vi "一体站单参数流程质控自动启动.vi"(6 "CODMn量程切换":enum32{"H", "L", "AUTO"}(ring)=enum."AUTO", 8 "总磷量程切换":enum32{"H", "L", "AUTO"}(ring)=enum."AUTO", 9 "总氮量程切换":enum32{"H", "L", "AUTO"}(ring)=enum."AUTO", 10 "氨氮量程切换":enum32{"H", "L", "AUTO"}(ring)=enum."AUTO", 11 "参数":T1={"是否启用仪器"=FALSE, "CODMn"={"启动测量模式"={"测量模式"=enum."水样测量"}, "确定按钮"=TRUE}, "启动模块"={"氨氮"=FALSE, "总磷"=FALSE, "总氮"=FALSE, "CODMn"=FALSE, "CODCr"=FALSE}, "常规启动"=FALSE, "直接启动"=FALSE}) -> ()   [LabVIEW 2016]
panel:
  out "枚举":enum16{"初始化", "采配水启动", "等待", "配水", "排水", "结束"}(ring)
  out "枚举 2":enum16{"初始化", "采配水启动", "等待", "配水", "排水", "结束"}(ring)
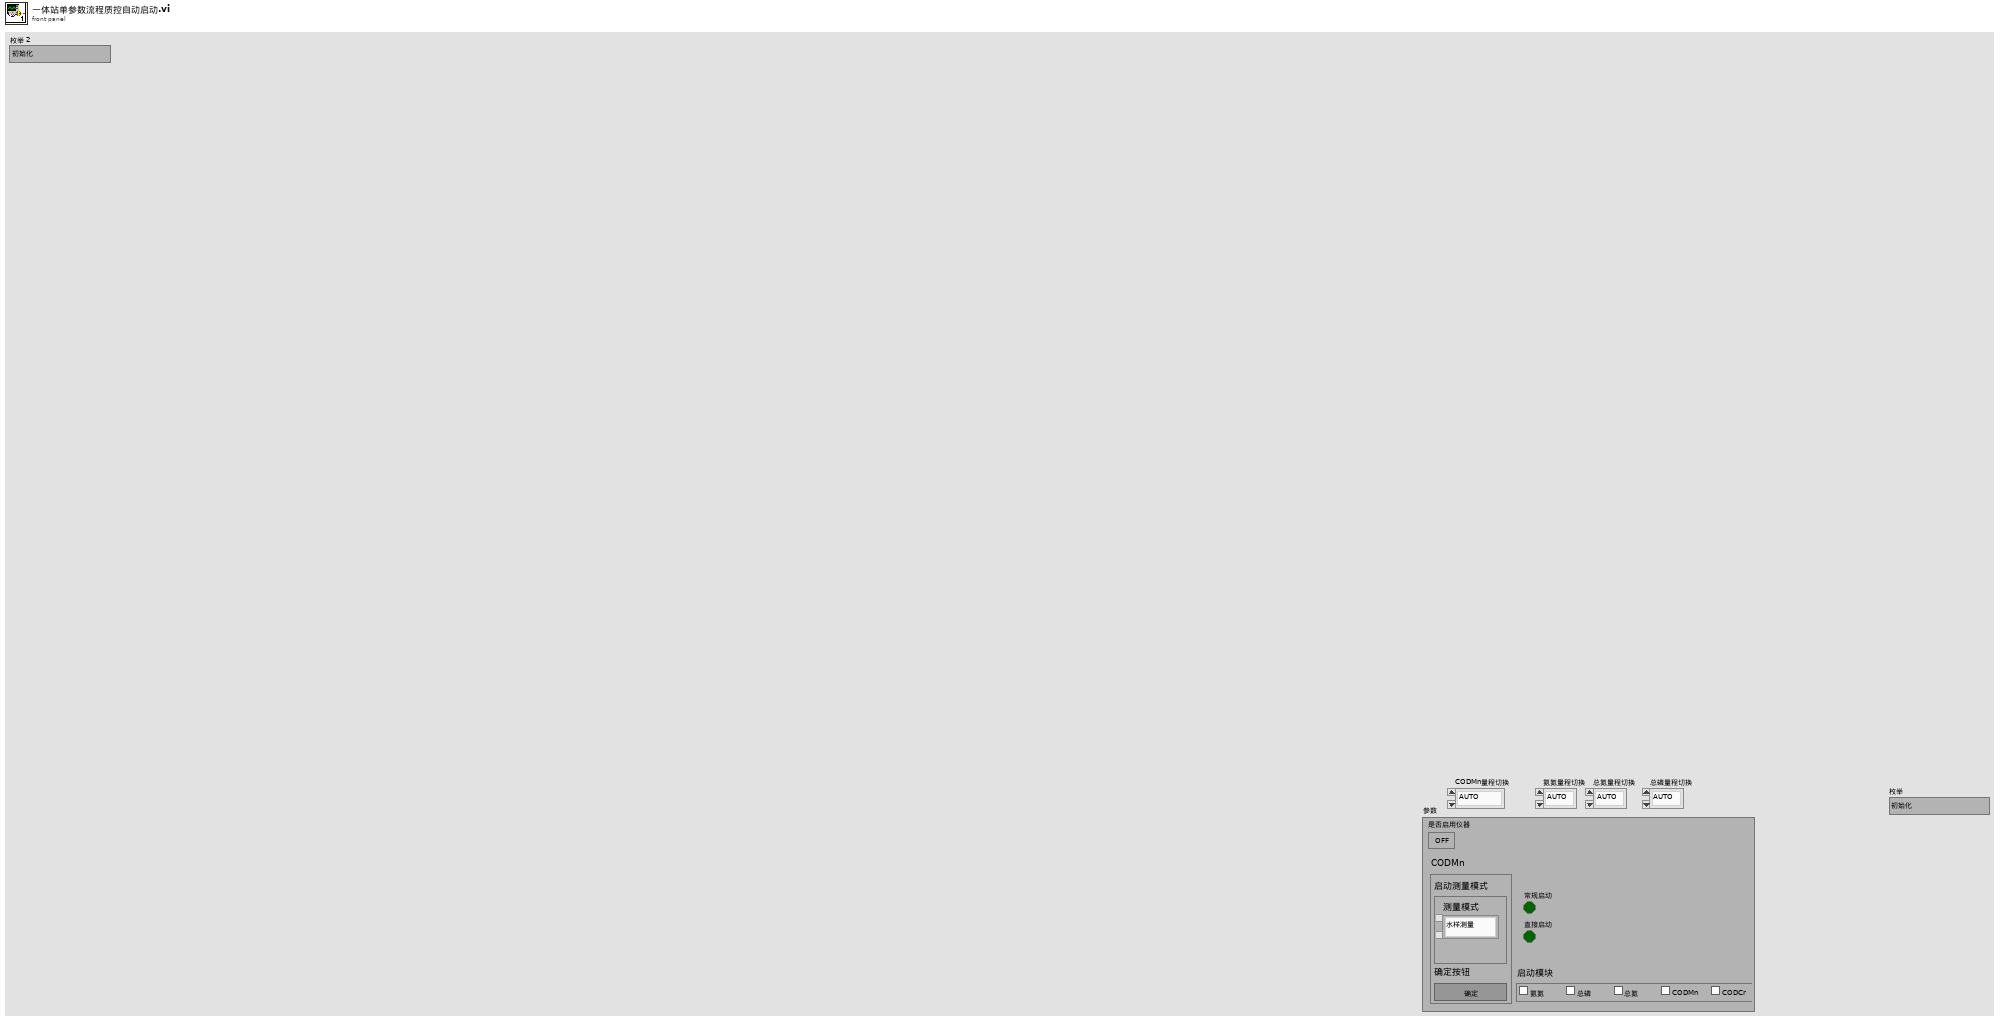
[diagram p1: front panel]
types:
  T1 = cluster{"是否启用仪器":bool, "CODMn":cluster{"启动测量模式":cluster{"测量模式":enum16{"水样测量", "标样核查", "加标回收", "平行样", "校零", "校标"}}, "确定按钮":bool}, "启动模块":cluster{"氨氮":bool, "总磷":bool, "总氮":bool, "CODMn":bool, "CODCr":bool}, "常规启动":bool, "直接启动":bool}
  T2 = cluster{"命令":string, cluster{"starting address":u16, "holding register value":u16}}
  T3 = cluster{"R0":i16, "R1":i16, "R2":i16, "R3":i16, "R4":i16, "R5":i16, "R6":i16, "R7":i16, "R8":i16, "R9":i16, "R10":i16, "R11":i16, "R12":i16, "R13":i16, "R14":i16, "R15":i16, "R16":i16, "R17":i16, "R18":i16, "R19":i16, "R20":i16, "R21":i16, "R22":i16, "R23":i16, "R24":i16, "R25":i16, "R26":i16, "R27":i16, "R28":i16, "R29":i16, "R30":i16, "R31":i16, "R32":i16, "R33":i16, "R34":i16, "R35":i16, "R36":i16, "R37":i16, "R38":i16, "R39":i16, "R40":i16, "R41":i16, "R42":i16, "R43":i16, "R44":i16, "R45":i16, "R46":i16, "R47":i16, "R48":i16, "R49":i16, "R50":i16, "R51":i16, "R52":i16, "R53":i16, "R54":i16, "R55":i16, "R56":i16}
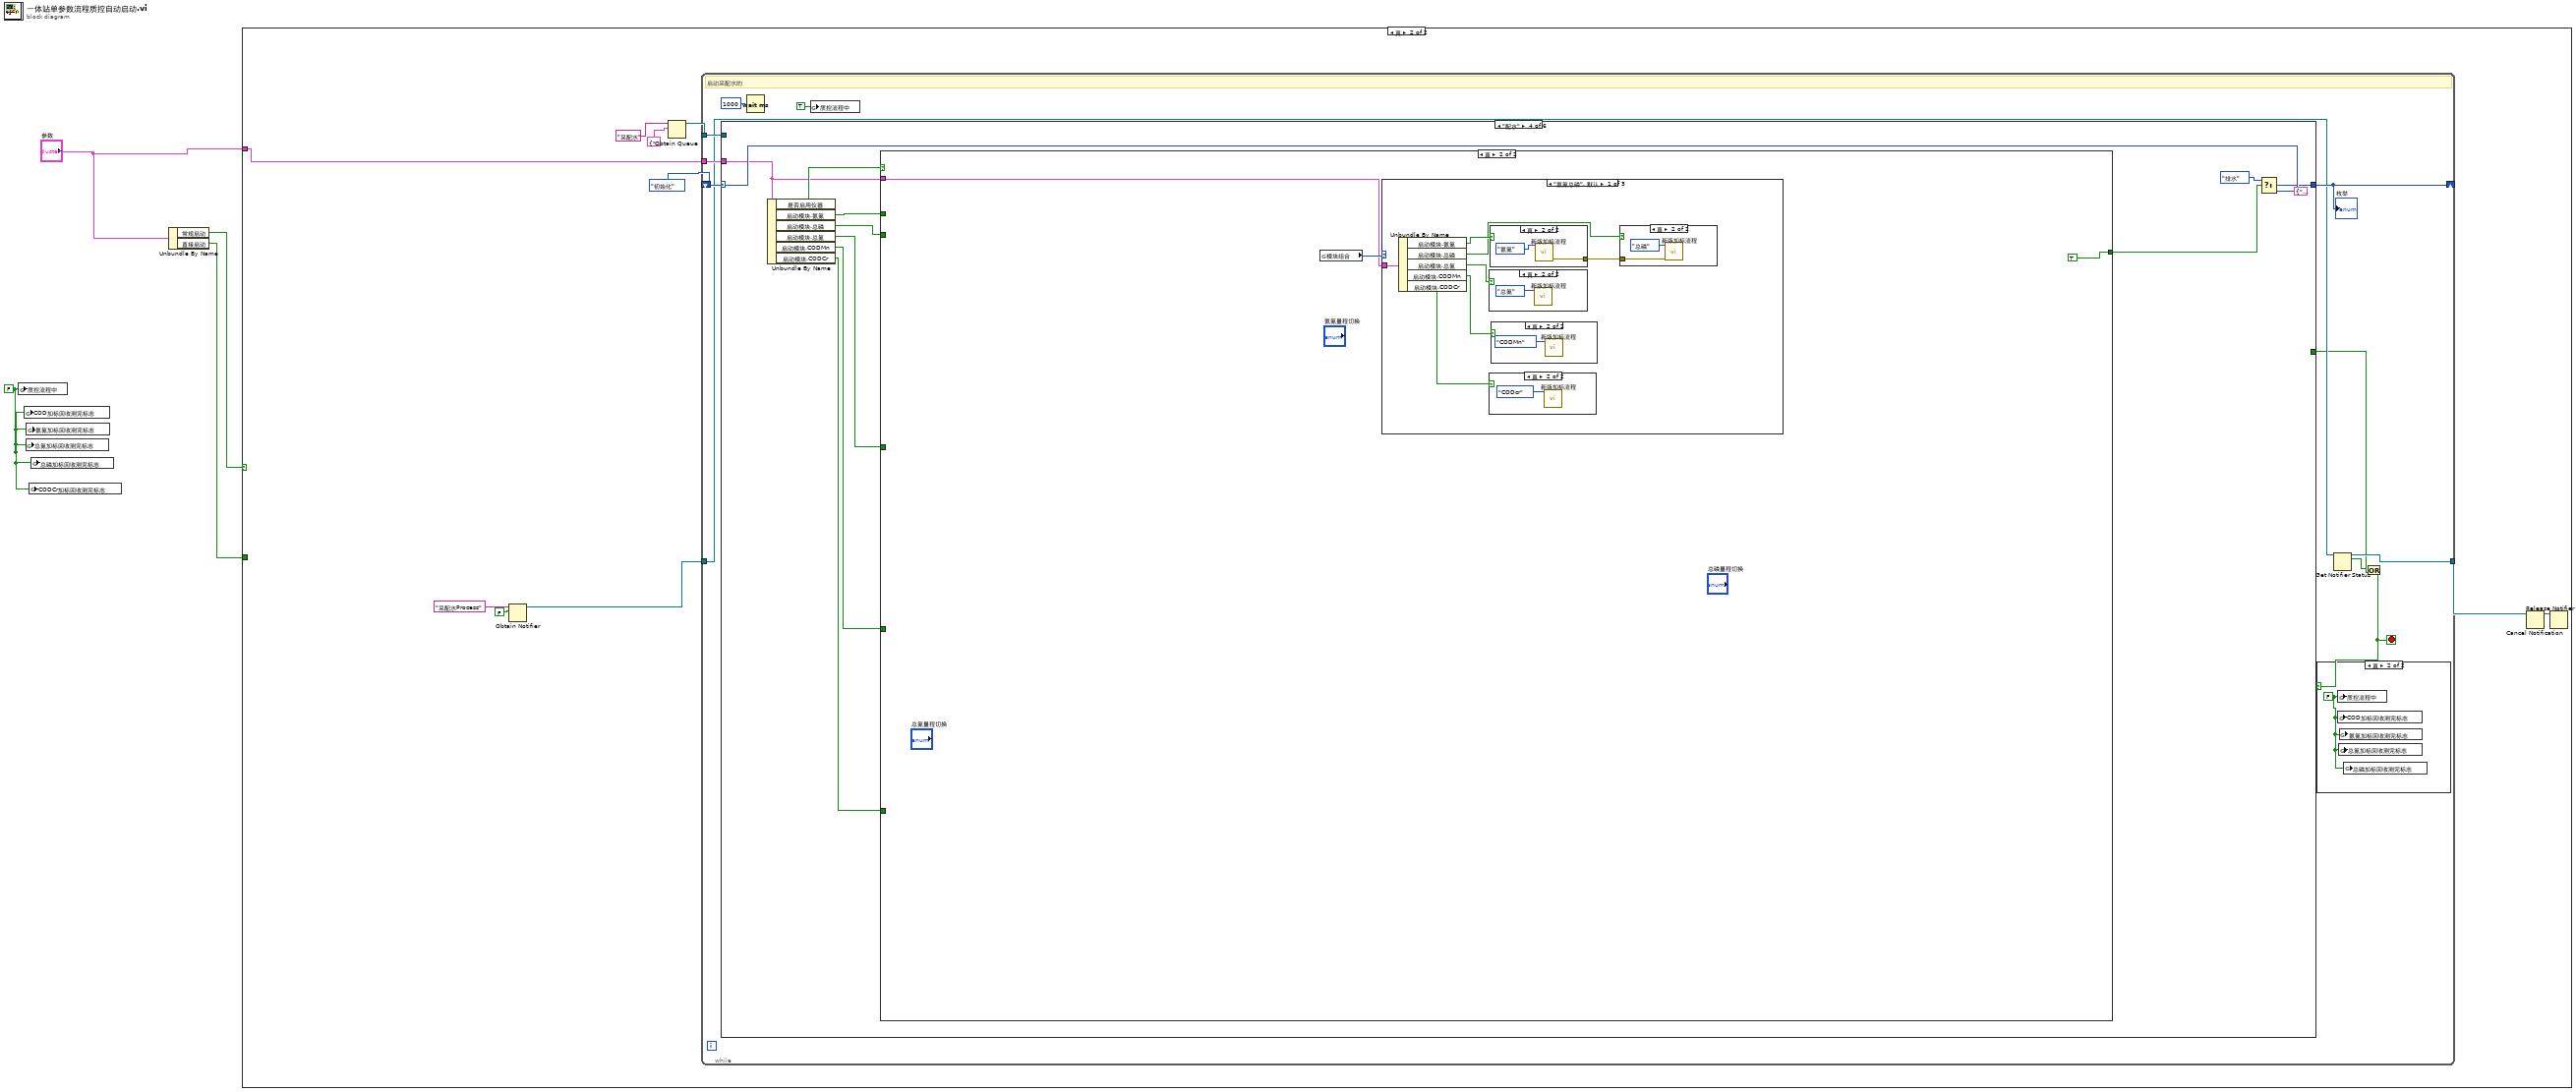
[diagram p0: block diagram]
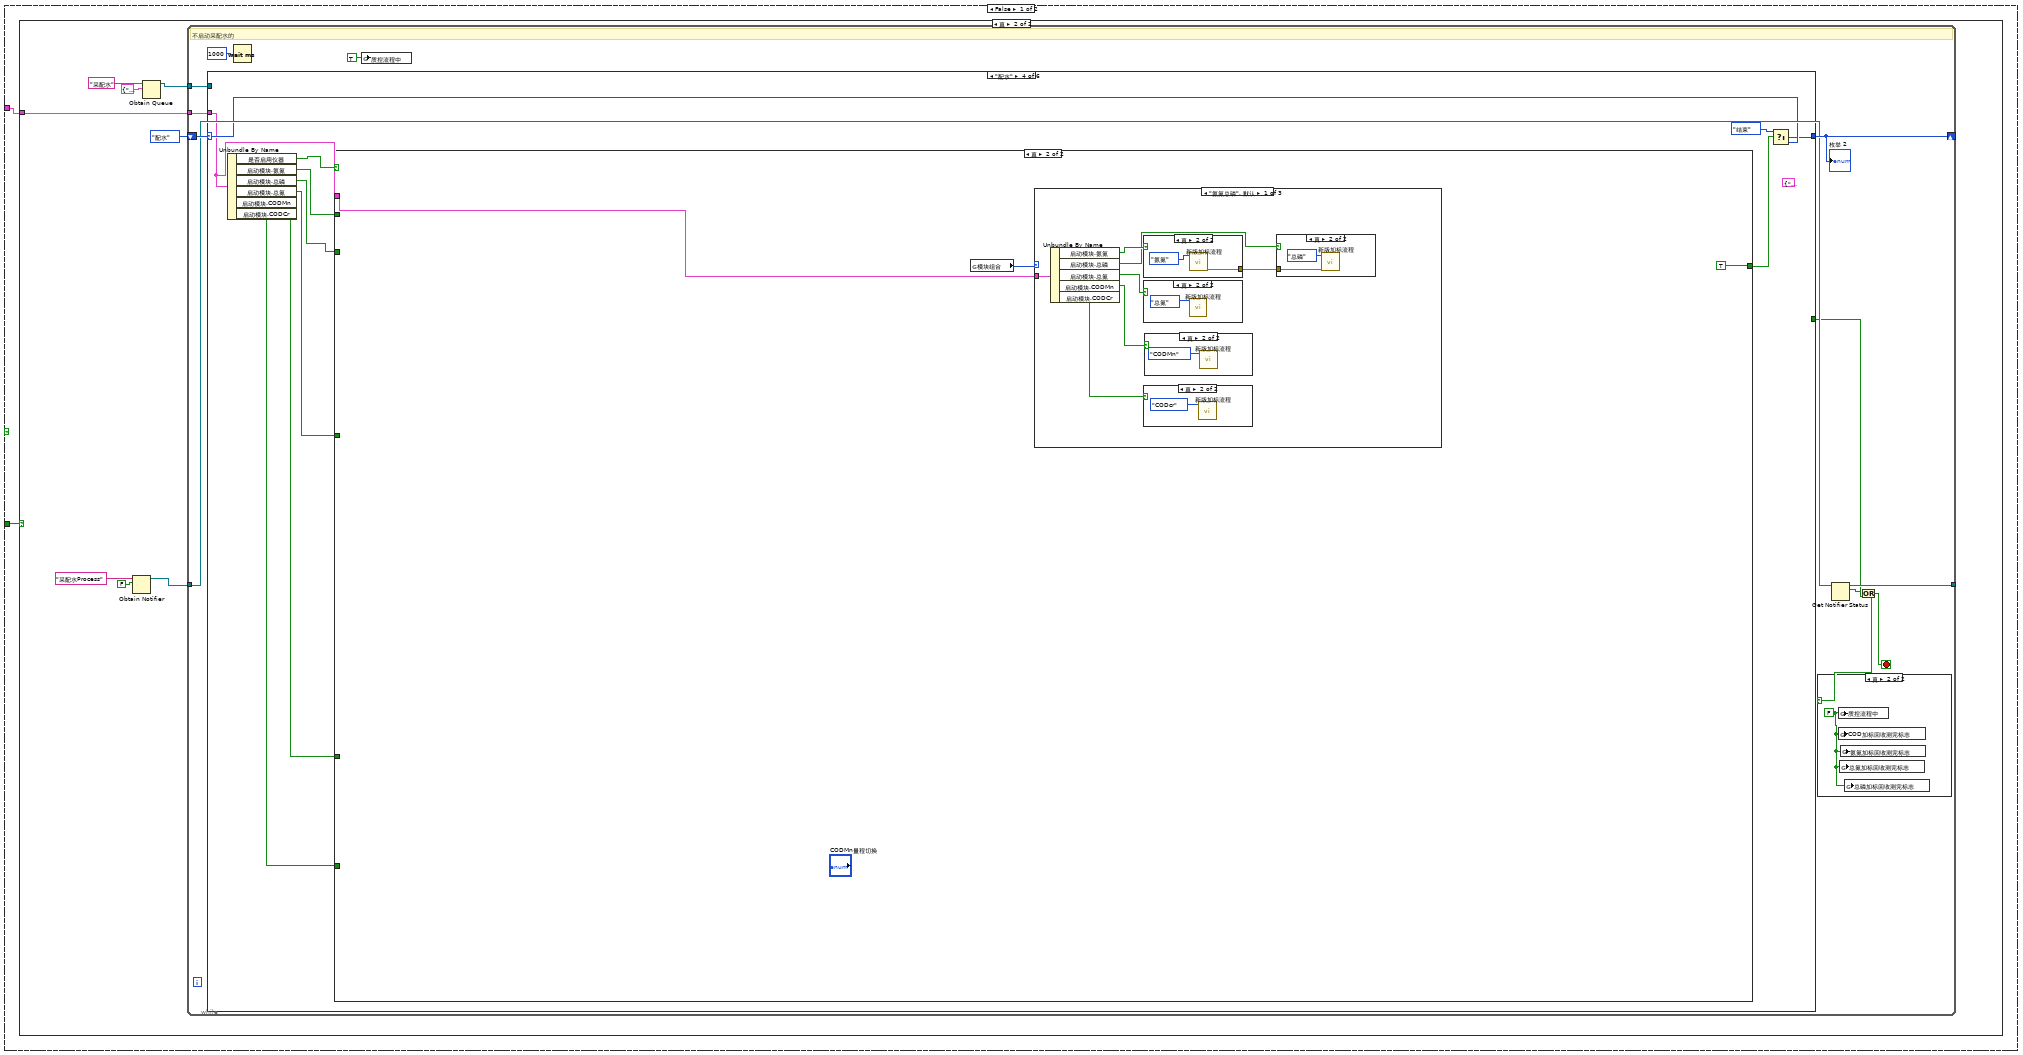
[diagram p2: hidden frame]
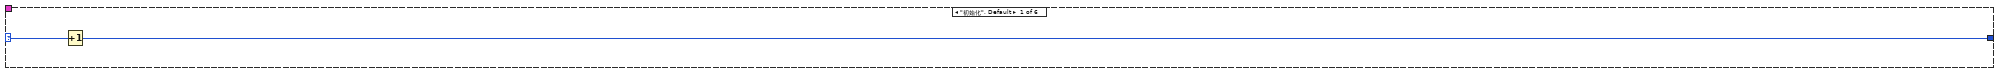
[diagram p5: hidden frame]
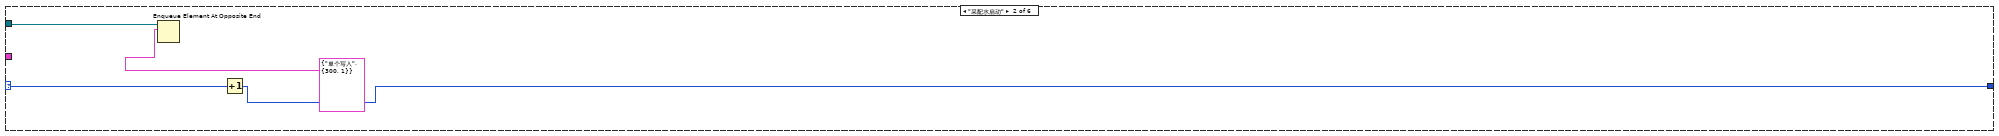
[diagram p6: hidden frame]
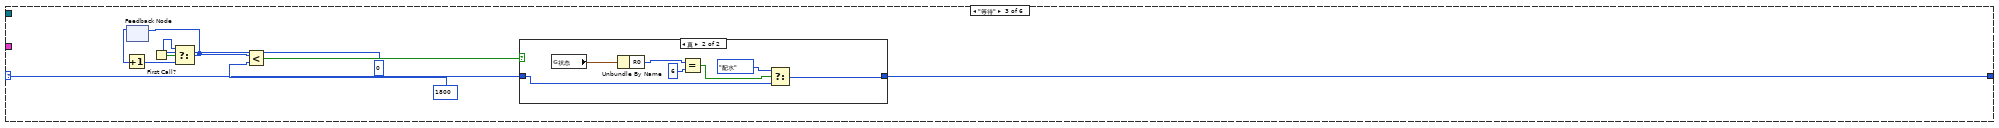
[diagram p7: hidden frame]
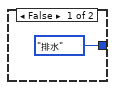
[diagram p8: hidden frame]
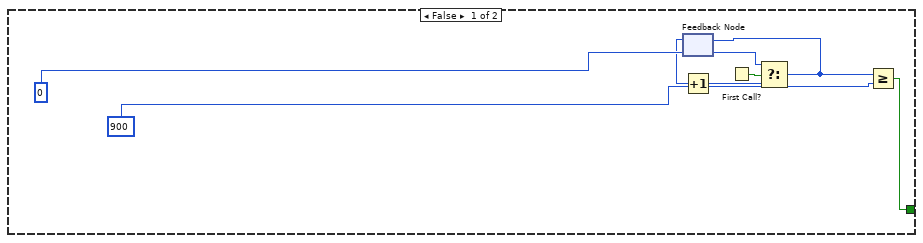
[diagram p9: hidden frame]
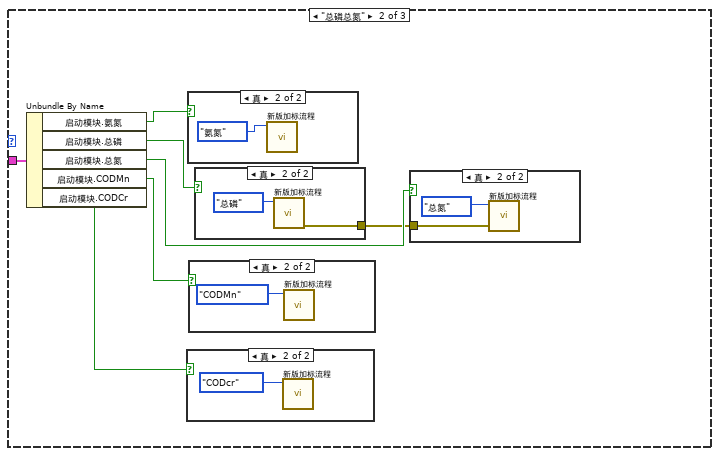
[diagram p15: hidden frame]
diagram:
  w1 = FALSE ("质控流程中")
  n1 = global write "质控测完标志全局 1.vi" "质控流程中"(w1) -> ()
  n2 = global write "质控测完标志全局 1.vi" "COD加标回收测完标志"(w1) -> ()
  n3 = global write "质控测完标志全局 1.vi" "总氮加标回收测完标志"(w1) -> ()
  n4 = global write "质控测完标志全局 1.vi" "氨氮加标回收测完标志"(w1) -> ()
  n5 = global write "质控测完标志全局 1.vi" "CODCr加标回收测完标志"(w1) -> ()
  n6 = global write "质控测完标志全局 1.vi" "总磷加标回收测完标志"(w1) -> ()
  n7 = Unbundle By Name("参数") -> ("常规启动"=w3:bool, "直接启动"=w2:bool)
  n8 = case shown="真" w3 {
    tunnel: "参数" -> [w5 w117]
    tunnel: w2 -> [w6 _]
    frame False {
      n9 = case shown="真" w6 {
        tunnel: w5 -> [_ w13]
        frame False {
        }
        frame True {
          n10 = Obtain Notifier(name (unnamed)="采配水Process" ("名称（未命名）"), notification data type=FALSE) -> (notifier out=w7:refnum<notifier>)  [unwired: 2 in, 2 out]
          n11 = Obtain Queue(name (unnamed)="采配水" ("名称（未命名）"), element data type=cluster{"命令":string, "数据":variant} {"命令"="", "数据"=variant}) -> (queue out=w10:refnum<queue>)  [unwired: 3 in, 2 out]
          n12 = while {
            tunnel: w10 -> [w25]
            shift-right: [w23] -> _
            shift-left: enum16{"初始化", "采配水启动", "等待", "配水", "排水", "结束"}."配水" ("枚举") -> [w24]
            tunnel: w13 -> [w21]
            tunnel: w7 -> [w20]
            tunnel: [w19] -> _
            stop <- w16 stop-if-true
            # "不启动采配水的"
            n13 = case shown="\"配水\"" w24 {
              selector: w24 -> [w28 w30 w39 w59 w111 w116]
              tunnel: w25 -> [_ w31 _ _ w112 _]
              tunnel: [w27 w29 w38 w58 w110 w115] -> w23
              tunnel: [_ _ _ _ _ TRUE] -> w18
              tunnel: w21 -> [_ _ _ w50 _ _]
              frame "初始化", Default {
                n14 = Increment(x=w28) -> (x+1=w27:enum16{"初始化", "采配水启动", "等待", "配水", "排水", "结束"})
              }
              frame "采配水启动" {
                n15 = Enqueue Element At Opposite End(queue=w31, element=T2 {"命令"="单个写入", {"starting address"=300, "holding register value"=1}} ("元素")) -> ()  [unwired: 2 in, 3 out]
                n16 = Increment(x=w30) -> (x+1=w29:enum16{"初始化", "采配水启动", "等待", "配水", "排水", "结束"})
              }
              frame "等待" {
                n17 = feedback #1() -> (w35:i32)  [unwired: 1 in]
                n18 = Increment(x=w35) -> (x+1=w34:i32)
                n19 = First Call?() -> (First Call?: T/F=w36:bool)
                n20 = Select(t=0, s=w36, f=w34) -> (s? t:f=w33:i32)
                n21 = feedback-in #1(w33) -> ()
                n22 = Less?(x=w33, y=1800) -> (x < y?=w40:bool)
                n23 = case shown="真" w40 {
                  tunnel: w39 -> [_ w45]
                  tunnel: [enum16{"初始化", "采配水启动", "等待", "配水", "排水", "结束"}."排水" ("枚举") w44] -> w38
                  frame False {
                  }
                  frame True {
                    n24 = global read "与采配水交互全局.vi" "状态"() -> (w43:T3)
                    n25 = Unbundle By Name(w43) -> ("R0"=w49:i16)
                    n26 = Equal?(x=w49, y=i16 6) -> (x = y?=w47:bool)
                    n27 = Select(t=enum16{"初始化", "采配水启动", "等待", "配水", "排水", "结束"}."配水" ("枚举"), s=w47, f=w45) -> (s? t:f=w44:enum16{"初始化", "采配水启动", "等待", "配水", "排水", "结束"})
                  }
                }
              }
              frame "配水" {
                (unwired) cluster{"命令":string, "data":variant} {"命令"="启动", "data"=variant(cluster{"站号":u16, "控制命令输出":u16[]} {"站号"=1, "控制命令输出"=[256, 0]})} ("元素")
                n28 = Unbundle By Name(w50) -> ("是否启用仪器"=w57:bool, "启动模块.氨氮"=w54:bool, "启动模块.总磷"=w55:bool, "启动模块.总氮"=w52:bool, "启动模块.CODMn"=w53:bool, "启动模块.CODCr"=w51:bool)
                n29 = case shown="真" w57 {
                  tunnel: [w61 TRUE] -> w56
                  tunnel: w55 -> [_ _]
                  tunnel: w54 -> [_ _]
                  tunnel: w53 -> [_ _]
                  tunnel: w52 -> [_ _]
                  tunnel: w51 -> [_ _]
                  tunnel: w50 -> [_ w69]
                  frame False {
                    n30 = feedback #2() -> (w65:i32)  [unwired: 1 in]
                    n31 = Increment(x=w65) -> (x+1=w64:i32)
                    n32 = First Call?() -> (First Call?: T/F=w66:bool)
                    n33 = Select(t=0, s=w66, f=w64) -> (s? t:f=w62:i32)
                    n34 = feedback-in #2(w62) -> ()
                    n35 = Greater Or Equal?(x=w62, y=900) -> (x >= y?=w61:bool)
                  }
                  frame True {
                    n36 = global read "断电保存全局.vi" "模块组合"() -> (w70:enum16{"氨氮总磷", "总磷总氮", "氨氮、总磷、总氮"})
                    n37 = case shown="\"氨氮总磷\", 默认" w70 {
                      tunnel: w69 -> [w77 w88 w104]
                      frame "氨氮总磷", Default {
                        n38 = Unbundle By Name(w77) -> ("启动模块.氨氮"=w76:bool, "启动模块.总磷"=w74:bool, "启动模块.总氮"=w73:bool, "启动模块.CODMn"=w72:bool, "启动模块.CODCr"=w71:bool)
                        n39 = case shown="真" w73 {
                          frame False {
                          }
                          frame True {
                            n40 = call "新版加标流程.vi"("参数"=enum16{"氨氮", "总磷", "总氮", "CODMn", "CODcr"}."总氮") -> ()  [unwired: 10 in, 1 out]
                          }
                        }
                        n41 = case shown="真" w71 {
                          frame False {
                          }
                          frame True {
                            n42 = call "新版加标流程.vi"("参数"=enum16{"氨氮", "总磷", "总氮", "CODMn", "CODcr"}."CODcr") -> ()  [unwired: 10 in, 1 out]
                          }
                        }
                        n43 = case shown="真" w76 {
                          tunnel: [_ w83] -> w75
                          frame False {
                          }
                          frame True {
                            n44 = call "新版加标流程.vi"("参数"=enum16{"氨氮", "总磷", "总氮", "CODMn", "CODcr"}."氨氮") -> ("error out"=w83:errorcluster)  [unwired: 10 in]
                          }
                        }
                        n45 = case shown="真" w72 {
                          frame False {
                          }
                          frame True {
                            n46 = call "新版加标流程.vi"("参数"=enum16{"氨氮", "总磷", "总氮", "CODMn", "CODcr"}."CODMn") -> ()  [unwired: 10 in, 1 out]
                          }
                        }
                        n47 = case shown="真" w74 {
                          tunnel: w75 -> [_ w81]
                          frame False {
                          }
                          frame True {
                            n48 = call "新版加标流程.vi"("error in (no error)"=w81, "参数"=enum16{"氨氮", "总磷", "总氮", "CODMn", "CODcr"}."总磷") -> ()  [unwired: 9 in, 1 out]
                          }
                        }
                      }
                      frame "总磷总氮" {
                        n49 = Unbundle By Name(w88) -> ("启动模块.氨氮"=w91:bool, "启动模块.总磷"=w87:bool, "启动模块.总氮"=w86:bool, "启动模块.CODMn"=w90:bool, "启动模块.CODCr"=w89:bool)
                        n50 = case shown="真" w89 {
                          frame False {
                          }
                          frame True {
                            n51 = call "新版加标流程.vi"("参数"=enum16{"氨氮", "总磷", "总氮", "CODMn", "CODcr"}."CODcr") -> ()  [unwired: 10 in, 1 out]
                          }
                        }
                        n52 = case shown="真" w91 {
                          frame False {
                          }
                          frame True {
                            n53 = call "新版加标流程.vi"("参数"=enum16{"氨氮", "总磷", "总氮", "CODMn", "CODcr"}."氨氮") -> ()  [unwired: 10 in, 1 out]
                          }
                        }
                        n54 = case shown="真" w90 {
                          frame False {
                          }
                          frame True {
                            n55 = call "新版加标流程.vi"("参数"=enum16{"氨氮", "总磷", "总氮", "CODMn", "CODcr"}."CODMn") -> ()  [unwired: 10 in, 1 out]
                          }
                        }
                        n56 = case shown="真" w87 {
                          tunnel: [_ w96] -> w85
                          frame False {
                          }
                          frame True {
                            n57 = call "新版加标流程.vi"("参数"=enum16{"氨氮", "总磷", "总氮", "CODMn", "CODcr"}."总磷") -> ("error out"=w96:errorcluster)  [unwired: 10 in]
                          }
                        }
                        n58 = case shown="真" w86 {
                          tunnel: w85 -> [_ w94]
                          frame False {
                          }
                          frame True {
                            n59 = call "新版加标流程.vi"("error in (no error)"=w94, "参数"=enum16{"氨氮", "总磷", "总氮", "CODMn", "CODcr"}."总氮") -> ()  [unwired: 9 in, 1 out]
                          }
                        }
                      }
                      frame "氨氮、总磷、总氮" {
                        n60 = Unbundle By Name(w104) -> ("启动模块.氨氮"=w103:bool, "启动模块.总磷"=w102:bool, "启动模块.总氮"=w101:bool, "启动模块.CODMn"=w99:bool, "启动模块.CODCr"=w100:bool)
                        n61 = case shown="真" w102 {
                          frame False {
                          }
                          frame True {
                            n62 = call "新版加标流程.vi"("参数"=enum16{"氨氮", "总磷", "总氮", "CODMn", "CODcr"}."总磷") -> ()  [unwired: 10 in, 1 out]
                          }
                        }
                        n63 = case shown="真" w101 {
                          frame False {
                          }
                          frame True {
                            n64 = call "新版加标流程.vi"("参数"=enum16{"氨氮", "总磷", "总氮", "CODMn", "CODcr"}."总氮") -> ()  [unwired: 10 in, 1 out]
                          }
                        }
                        n65 = case shown="真" w103 {
                          frame False {
                          }
                          frame True {
                            n66 = call "新版加标流程.vi"("参数"=enum16{"氨氮", "总磷", "总氮", "CODMn", "CODcr"}."氨氮") -> ()  [unwired: 10 in, 1 out]
                          }
                        }
                        n67 = case shown="真" w99 {
                          frame False {
                          }
                          frame True {
                            n68 = call "新版加标流程.vi"("参数"=enum16{"氨氮", "总磷", "总氮", "CODMn", "CODcr"}."CODMn") -> ()  [unwired: 10 in, 1 out]
                          }
                        }
                        n69 = case shown="真" w100 {
                          frame False {
                          }
                          frame True {
                            n70 = call "新版加标流程.vi"("参数"=enum16{"氨氮", "总磷", "总氮", "CODMn", "CODcr"}."CODcr") -> ()  [unwired: 10 in, 1 out]
                          }
                        }
                      }
                    }
                  }
                }
                n71 = Select(t=enum16{"初始化", "采配水启动", "等待", "配水", "排水", "结束"}."结束" ("枚举"), s=w56, f=w59) -> (s? t:f=w58:enum16{"初始化", "采配水启动", "等待", "配水", "排水", "结束"})
              }
              frame "排水" {
                n72 = Enqueue Element At Opposite End(queue=w112, element=T2 {"命令"="单个写入", {"starting address"=303, "holding register value"=1}} ("元素")) -> ()  [unwired: 2 in, 3 out]
                n73 = Increment(x=w111) -> (x+1=w110:enum16{"初始化", "采配水启动", "等待", "配水", "排水", "结束"})
              }
              frame "结束" {
                n74 = Increment(x=w116) -> (x+1=w115:enum16{"初始化", "采配水启动", "等待", "配水", "排水", "结束"})
              }
            }
            "枚举 2" <- w23
            n75 = Wait (ms)(milliseconds to wait=u32 1000 ("等待时间（毫秒）")) -> ()  [unwired: 1 out]
            n76 = global write "质控测完标志全局 1.vi" "质控流程中"(TRUE ("质控流程中")) -> ()
            n77 = Get Notifier Status(notifier=w20) -> (notifier out=w19:refnum<notifier>, current notification=w17:bool)  [unwired: 1 in, 3 out]
            n78 = Or(x=w17, y=w18) -> (x .or. y?=w16:bool)
            n79 = case shown="真" w16 {
              frame False {
              }
              frame True {
                w26 = FALSE ("质控流程中")
                n80 = global write "质控测完标志全局 1.vi" "质控流程中"(w26) -> ()
                n81 = global write "质控测完标志全局 1.vi" "COD加标回收测完标志"(w26) -> ()
                n82 = global write "质控测完标志全局 1.vi" "总氮加标回收测完标志"(w26) -> ()
                n83 = global write "质控测完标志全局 1.vi" "氨氮加标回收测完标志"(w26) -> ()
                n84 = global write "质控测完标志全局 1.vi" "总磷加标回收测完标志"(w26) -> ()
              }
            }
          }
        }
      }
    }
    frame True {
      n85 = Obtain Notifier(name (unnamed)="采配水Process" ("名称（未命名）"), notification data type=FALSE) -> (notifier out=w120:refnum<notifier>)  [unwired: 2 in, 2 out]
      n86 = Obtain Queue(name (unnamed)="采配水" ("名称（未命名）"), element data type=cluster{"命令":string, "数据":variant} {"命令"="", "数据"=variant}) -> (queue out=w124:refnum<queue>)  [unwired: 3 in, 2 out]
      n87 = while {
        tunnel: w124 -> [w137]
        shift-right: [w135] -> _
        shift-left: enum16{"初始化", "采配水启动", "等待", "配水", "排水", "结束"}."初始化" ("枚举") -> [w136]
        tunnel: w117 -> [w133]
        tunnel: w120 -> [w132]
        tunnel: [w131] -> w119
        stop <- w128 stop-if-true
        # "启动采配水的"
        n88 = case shown="\"配水\"" w136 {
          selector: w136 -> [w140 w144 w153 w173 w225 w230]
          tunnel: w137 -> [_ w145 _ _ w226 _]
          tunnel: [w139 w143 w152 w172 w224 w229] -> w135
          tunnel: [_ _ _ _ _ TRUE] -> w130
          tunnel: w133 -> [_ _ _ w164 _ _]
          frame "初始化", Default {
            n89 = Increment(x=w140) -> (x+1=w139:enum16{"初始化", "采配水启动", "等待", "配水", "排水", "结束"})
          }
          frame "采配水启动" {
            n90 = Enqueue Element At Opposite End(queue=w145, element=T2 {"命令"="单个写入", {"starting address"=300, "holding register value"=1}} ("元素")) -> (queue out=w141:refnum<queue>)  [unwired: 2 in, 2 out]
            n91 = Increment(x=w144) -> (x+1=w143:enum16{"初始化", "采配水启动", "等待", "配水", "排水", "结束"})
            n92 = Enqueue Element At Opposite End(queue=w141, element=T2 {"命令"="单个写入", {"starting address"=303, "holding register value"=1}} ("元素")) -> ()  [unwired: 2 in, 3 out]
          }
          frame "等待" {
            n93 = feedback #3() -> (w149:i32)  [unwired: 1 in]
            n94 = Increment(x=w149) -> (x+1=w148:i32)
            n95 = First Call?() -> (First Call?: T/F=w150:bool)
            n96 = Select(t=0, s=w150, f=w148) -> (s? t:f=w147:i32)
            n97 = feedback-in #3(w147) -> ()
            n98 = Less?(x=w147, y=1800) -> (x < y?=w154:bool)
            n99 = case shown="真" w154 {
              tunnel: w153 -> [_ w159]
              tunnel: [enum16{"初始化", "采配水启动", "等待", "配水", "排水", "结束"}."排水" ("枚举") w158] -> w152
              frame False {
              }
              frame True {
                n100 = global read "与采配水交互全局.vi" "状态"() -> (w157:T3)
                n101 = Unbundle By Name(w157) -> ("R0"=w163:i16)
                n102 = Equal?(x=w163, y=i16 6) -> (x = y?=w161:bool)
                n103 = Select(t=enum16{"初始化", "采配水启动", "等待", "配水", "排水", "结束"}."配水" ("枚举"), s=w161, f=w159) -> (s? t:f=w158:enum16{"初始化", "采配水启动", "等待", "配水", "排水", "结束"})
              }
            }
          }
          frame "配水" {
            (unwired) cluster{"命令":string, "data":variant} {"命令"="启动", "data"=variant(cluster{"站号":u16, "控制命令输出":u16[]} {"站号"=1, "控制命令输出"=[256, 0]})} ("元素")
            n104 = Unbundle By Name(w164) -> ("是否启用仪器"=w171:bool, "启动模块.氨氮"=w168:bool, "启动模块.总磷"=w169:bool, "启动模块.总氮"=w166:bool, "启动模块.CODMn"=w167:bool, "启动模块.CODCr"=w165:bool)
            n105 = case shown="真" w171 {
              tunnel: [w175 TRUE] -> w170
              tunnel: w169 -> [_ _]
              tunnel: w168 -> [_ _]
              tunnel: w167 -> [_ _]
              tunnel: w166 -> [_ _]
              tunnel: w165 -> [_ _]
              tunnel: w164 -> [_ w183]
              frame False {
                n106 = feedback #4() -> (w179:i32)  [unwired: 1 in]
                n107 = Increment(x=w179) -> (x+1=w178:i32)
                n108 = First Call?() -> (First Call?: T/F=w180:bool)
                n109 = Select(t=0, s=w180, f=w178) -> (s? t:f=w176:i32)
                n110 = feedback-in #4(w176) -> ()
                n111 = Greater Or Equal?(x=w176, y=900) -> (x >= y?=w175:bool)
              }
              frame True {
                n112 = global read "断电保存全局.vi" "模块组合"() -> (w184:enum16{"氨氮总磷", "总磷总氮", "氨氮、总磷、总氮"})
                n113 = case shown="\"氨氮总磷\", 默认" w184 {
                  tunnel: w183 -> [w191 w202 w218]
                  frame "氨氮总磷", Default {
                    n114 = Unbundle By Name(w191) -> ("启动模块.氨氮"=w190:bool, "启动模块.总磷"=w188:bool, "启动模块.总氮"=w187:bool, "启动模块.CODMn"=w186:bool, "启动模块.CODCr"=w185:bool)
                    n115 = case shown="真" w187 {
                      frame False {
                      }
                      frame True {
                        n116 = call "新版加标流程.vi"("参数"=enum16{"氨氮", "总磷", "总氮", "CODMn", "CODcr"}."总氮") -> ()  [unwired: 10 in, 1 out]
                      }
                    }
                    n117 = case shown="真" w185 {
                      frame False {
                      }
                      frame True {
                        n118 = call "新版加标流程.vi"("参数"=enum16{"氨氮", "总磷", "总氮", "CODMn", "CODcr"}."CODcr") -> ()  [unwired: 10 in, 1 out]
                      }
                    }
                    n119 = case shown="真" w190 {
                      tunnel: [_ w197] -> w189
                      frame False {
                      }
                      frame True {
                        n120 = call "新版加标流程.vi"("参数"=enum16{"氨氮", "总磷", "总氮", "CODMn", "CODcr"}."氨氮") -> ("error out"=w197:errorcluster)  [unwired: 10 in]
                      }
                    }
                    n121 = case shown="真" w186 {
                      frame False {
                      }
                      frame True {
                        n122 = call "新版加标流程.vi"("参数"=enum16{"氨氮", "总磷", "总氮", "CODMn", "CODcr"}."CODMn") -> ()  [unwired: 10 in, 1 out]
                      }
                    }
                    n123 = case shown="真" w188 {
                      tunnel: w189 -> [_ w195]
                      frame False {
                      }
                      frame True {
                        n124 = call "新版加标流程.vi"("error in (no error)"=w195, "参数"=enum16{"氨氮", "总磷", "总氮", "CODMn", "CODcr"}."总磷") -> ()  [unwired: 9 in, 1 out]
                      }
                    }
                  }
                  frame "总磷总氮" {
                    n125 = Unbundle By Name(w202) -> ("启动模块.氨氮"=w205:bool, "启动模块.总磷"=w201:bool, "启动模块.总氮"=w200:bool, "启动模块.CODMn"=w204:bool, "启动模块.CODCr"=w203:bool)
                    n126 = case shown="真" w203 {
                      frame False {
                      }
                      frame True {
                        n127 = call "新版加标流程.vi"("参数"=enum16{"氨氮", "总磷", "总氮", "CODMn", "CODcr"}."CODcr") -> ()  [unwired: 10 in, 1 out]
                      }
                    }
                    n128 = case shown="真" w205 {
                      frame False {
                      }
                      frame True {
                        n129 = call "新版加标流程.vi"("参数"=enum16{"氨氮", "总磷", "总氮", "CODMn", "CODcr"}."氨氮") -> ()  [unwired: 10 in, 1 out]
                      }
                    }
                    n130 = case shown="真" w204 {
                      frame False {
                      }
                      frame True {
                        n131 = call "新版加标流程.vi"("参数"=enum16{"氨氮", "总磷", "总氮", "CODMn", "CODcr"}."CODMn") -> ()  [unwired: 10 in, 1 out]
                      }
                    }
                    n132 = case shown="真" w201 {
                      tunnel: [_ w210] -> w199
                      frame False {
                      }
                      frame True {
                        n133 = call "新版加标流程.vi"("参数"=enum16{"氨氮", "总磷", "总氮", "CODMn", "CODcr"}."总磷") -> ("error out"=w210:errorcluster)  [unwired: 10 in]
                      }
                    }
                    n134 = case shown="真" w200 {
                      tunnel: w199 -> [_ w208]
                      frame False {
                      }
                      frame True {
                        n135 = call "新版加标流程.vi"("error in (no error)"=w208, "参数"=enum16{"氨氮", "总磷", "总氮", "CODMn", "CODcr"}."总氮") -> ()  [unwired: 9 in, 1 out]
                      }
                    }
                  }
                  frame "氨氮、总磷、总氮" {
                    n136 = Unbundle By Name(w218) -> ("启动模块.氨氮"=w217:bool, "启动模块.总磷"=w216:bool, "启动模块.总氮"=w215:bool, "启动模块.CODMn"=w213:bool, "启动模块.CODCr"=w214:bool)
                    n137 = case shown="真" w216 {
                      frame False {
                      }
                      frame True {
                        n138 = call "新版加标流程.vi"("参数"=enum16{"氨氮", "总磷", "总氮", "CODMn", "CODcr"}."总磷") -> ()  [unwired: 10 in, 1 out]
                      }
                    }
                    n139 = case shown="真" w215 {
                      frame False {
                      }
                      frame True {
                        n140 = call "新版加标流程.vi"("参数"=enum16{"氨氮", "总磷", "总氮", "CODMn", "CODcr"}."总氮") -> ()  [unwired: 10 in, 1 out]
                      }
                    }
                    n141 = case shown="真" w217 {
                      frame False {
                      }
                      frame True {
                        n142 = call "新版加标流程.vi"("参数"=enum16{"氨氮", "总磷", "总氮", "CODMn", "CODcr"}."氨氮") -> ()  [unwired: 10 in, 1 out]
                      }
                    }
                    n143 = case shown="真" w213 {
                      frame False {
                      }
                      frame True {
                        n144 = call "新版加标流程.vi"("参数"=enum16{"氨氮", "总磷", "总氮", "CODMn", "CODcr"}."CODMn") -> ()  [unwired: 10 in, 1 out]
                      }
                    }
                    n145 = case shown="真" w214 {
                      frame False {
                      }
                      frame True {
                        n146 = call "新版加标流程.vi"("参数"=enum16{"氨氮", "总磷", "总氮", "CODMn", "CODcr"}."CODcr") -> ()  [unwired: 10 in, 1 out]
                      }
                    }
                  }
                }
              }
            }
            n147 = Select(t=enum16{"初始化", "采配水启动", "等待", "配水", "排水", "结束"}."排水" ("枚举"), s=w170, f=w173) -> (s? t:f=w172:enum16{"初始化", "采配水启动", "等待", "配水", "排水", "结束"})
          }
          frame "排水" {
            n148 = Enqueue Element At Opposite End(queue=w226, element=T2 {"命令"="单个写入", {"starting address"=303, "holding register value"=1}} ("元素")) -> ()  [unwired: 2 in, 3 out]
            n149 = Increment(x=w225) -> (x+1=w224:enum16{"初始化", "采配水启动", "等待", "配水", "排水", "结束"})
          }
          frame "结束" {
            n150 = Increment(x=w230) -> (x+1=w229:enum16{"初始化", "采配水启动", "等待", "配水", "排水", "结束"})
          }
        }
        "枚举" <- w135
        n151 = Wait (ms)(milliseconds to wait=u32 1000 ("等待时间（毫秒）")) -> ()  [unwired: 1 out]
        n152 = global write "质控测完标志全局 1.vi" "质控流程中"(TRUE ("质控流程中")) -> ()
        n153 = Get Notifier Status(notifier=w132) -> (notifier out=w131:refnum<notifier>, current notification=w129:bool)  [unwired: 1 in, 3 out]
        n154 = Or(x=w129, y=w130) -> (x .or. y?=w128:bool)
        n155 = case shown="真" w128 {
          frame False {
          }
          frame True {
            w138 = FALSE ("质控流程中")
            n156 = global write "质控测完标志全局 1.vi" "质控流程中"(w138) -> ()
            n157 = global write "质控测完标志全局 1.vi" "COD加标回收测完标志"(w138) -> ()
            n158 = global write "质控测完标志全局 1.vi" "总氮加标回收测完标志"(w138) -> ()
            n159 = global write "质控测完标志全局 1.vi" "氨氮加标回收测完标志"(w138) -> ()
            n160 = global write "质控测完标志全局 1.vi" "总磷加标回收测完标志"(w138) -> ()
          }
        }
      }
      n161 = Cancel Notification(0:w119) -> (8:w118:refnum<notifier>)  [unwired: 1 in, 2 out]
      n162 = Release Notifier(notifier=w118) -> ()  [unwired: 2 in, 3 out]
    }
  }
